vi "Spy Flush Last Call.vi"(8 "error in (no error)":errorcluster, 11 "Mock Process In":refnum<class "Mock Process.lvclass">) -> (0 "error out":errorcluster, 1 "Message Data":variant, 2 "Message":string, 3 "Mock Process Out":refnum<class "Mock Process.lvclass">)   [LabVIEW 2020, in "Mock Process.lvclass"]
doc: "Spys on errors sent to the error handler. This Method requires a lock on the execution thread to prevent race conditions when testing other processes using the error handler."
uses:
  Mock Process.lvclass
  Mock Process.lvclass/Mock Process.ctl
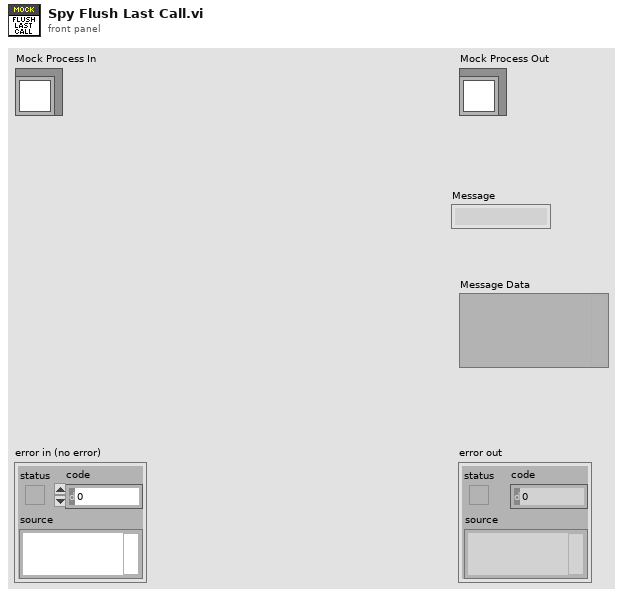
[diagram p1: front panel]
types:
  T1 = cluster{"Message":string, "Message Data":variant}[]
  T2 = cluster{"Message":string, "Message Data":variant}
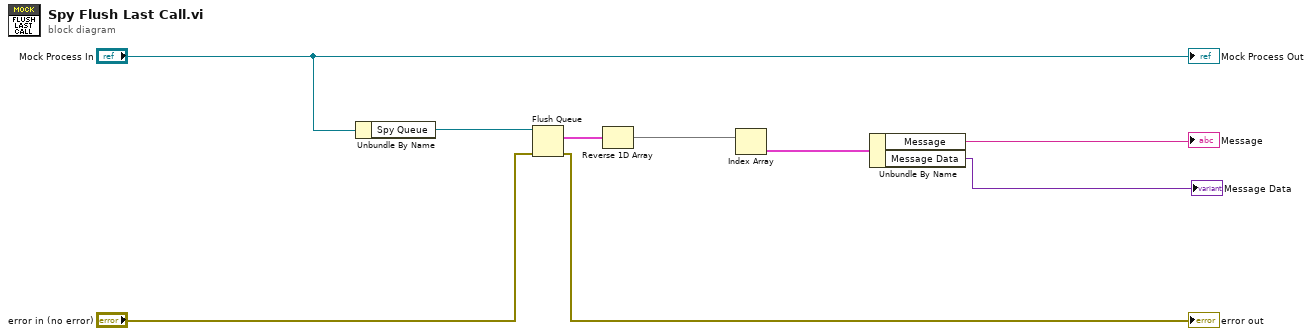
[diagram p0: block diagram]
diagram:
  n1 = Unbundle By Name("Mock Process In") -> ("Spy Queue"=w8:refnum<queue>)
  n2 = Flush Queue(queue=w8, error in (no error)="error in (no error)") -> (remaining elements=w6:T1, error out=→"error out":errorcluster)  [unwired: 1 out]
  n3 = Reverse 1D Array(array=w6) -> (reversed array=w3:T1)
  n4 = Index Array(array=w3) -> (element=w1:T2)  [unwired: 1 in]
  n5 = Unbundle By Name(w1) -> ("Message"=→"Message":string, "Message Data"=→"Message Data":variant)
  "Mock Process Out" <- "Mock Process In"
